vi "test dll.vi"() -> ()   [LabVIEW 2019]
panel:
  out "return type":i32
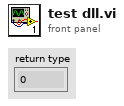
[diagram p1: front panel]
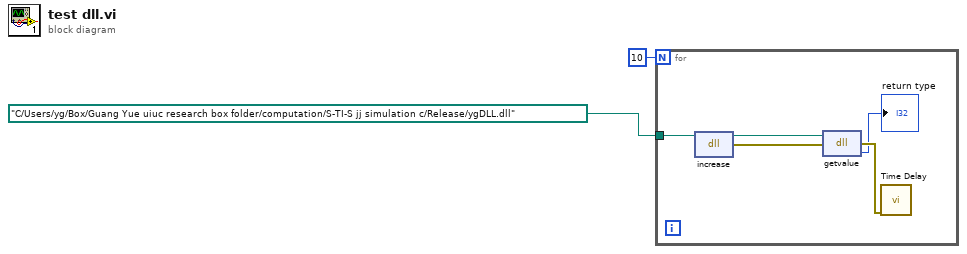
[diagram p0: block diagram]
diagram:
  n1 = for {
    N: 10 -> [_]
    tunnel: path "C:/Users/yg/Box/Guang Yue uiuc research box folder/computation/S-TI-S jj simulation c/Release/ygDLL.dll" ("path in") -> [w6]
    n2 = dll-call lib="C:/Users/yg/Box/Guang Yue uiuc research box folder/computation/S-TI-S jj simulation c/Release/ygDLL.dll" fn="increase"(path in=w6) -> (path out=w5:path, error out=w7:errorcluster)  [unwired: 3 in]
    n3 = dll-call lib="C:/Users/yg/Box/Guang Yue uiuc research box folder/computation/S-TI-S jj simulation c/Release/ygDLL.dll" fn="getvalue"(path in=w5, error in=w7) -> (error out=w4:errorcluster, "return type"=→"return type":i32)  [unwired: 1 in, 1 out]
    n4 = call "Time Delay"("error in (no error)"=w4) -> ()  [unwired: 10 in, 1 out]
  }
